vi "stageWaitForStandby.vi"(10 "error in":errorcluster, 11 "VISA resource name in":refnum<visa-resource-name>) -> (2 "error out":errorcluster, 3 "VISA resource name out 2":refnum<visa-resource-name>)   [LabVIEW 2016]
uses:
  variables/applicationControl.vi
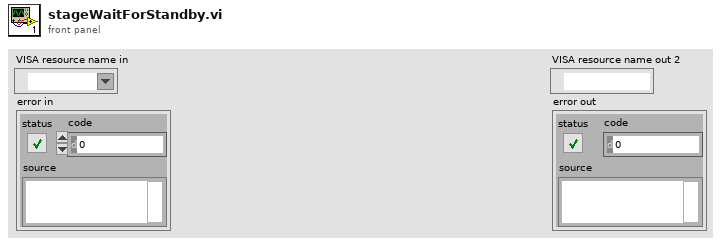
[diagram p1: front panel]
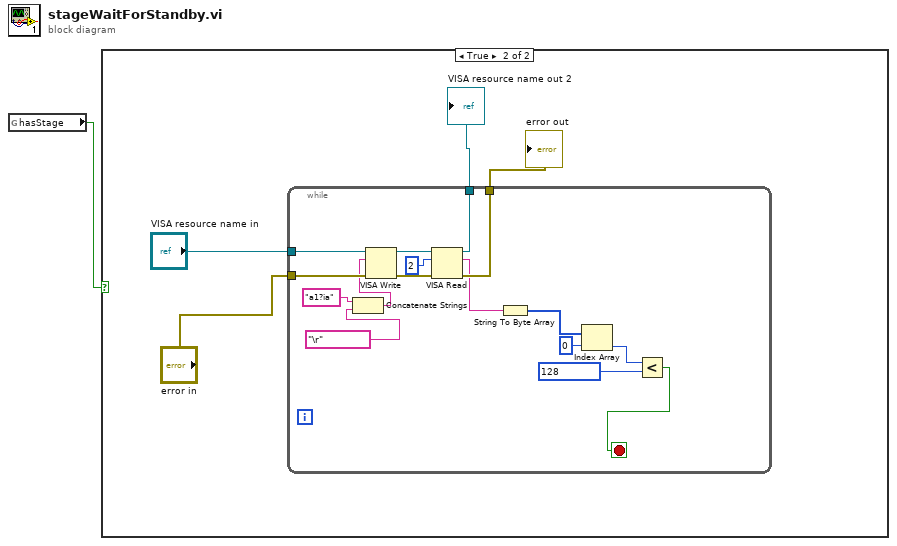
[diagram p0: block diagram]
diagram:
  n1 = global read "applicationControl.vi" "hasStage"() -> (w1:bool)
  n2 = case shown="True" w1 {
    frame False {
    }
    frame True {
      n3 = while {
        tunnel: "VISA resource name in" -> [w21]
        tunnel: "error in" -> [w20]
        tunnel: [w13] -> w3
        tunnel: [w12] -> w2
        stop <- w6 stop-if-true
        n4 = Concatenate Strings("a1?ia" ("write buffer"), "\r" ("write buffer")) -> (w17:string)
        n5 = VISA Write(VISA resource name=w21, write buffer=w17, error in (no error)=w20) -> (VISA resource name out=w16:refnum<visa-resource-name>, error out=w15:errorcluster)  [unwired: 1 out]
        n6 = VISA Read(VISA resource name=w16, byte count=u32 2, error in (no error)=w15) -> (VISA resource name out=w13:refnum<visa-resource-name>, read buffer=w11:string, error out=w12:errorcluster)  [unwired: 1 out]
        n7 = String To Byte Array(string=w11) -> (unsigned byte array=w10:u8[])
        n8 = Index Array(array=w10, index=0) -> (element=w8:u8)
        n9 = Less?(x=w8, y=u8 128) -> (x < y?=w6:bool)
      }
      "VISA resource name out 2" <- w3
      "error out" <- w2
    }
  }
